vi "driveCheesy.vi"() -> ()   [LabVIEW 2012]
uses:
  <vilib>/Utility/inputDevices.llb/joystickAcquire.vi
panel:
  in  "low gear drive constant slow":dbl
  in  "low gear drive constant fast":dbl
  in  "Gear":bool
  in  "high gear drive constant slow":dbl
  in  "high gear drive constant fast":dbl
  in  "y axis":dbl
  in  "z axis":dbl
  out "Right Side Motors":dbl
  out "Left Side Motors":dbl
  # "High"
  # "Low"
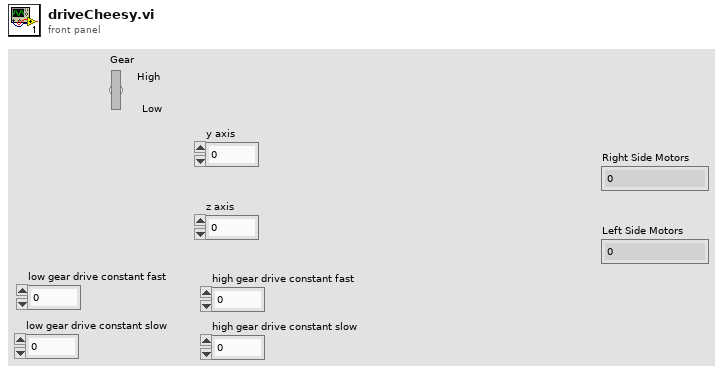
[diagram p1: front panel]
types:
  T1 = cluster{"X axis":i32, "Y axis":i32, "Z axis":i32, "X axis rotation":i32, "Y axis rotation":i32, "Z axis rotation":i32, "U axis":i32, "V axis":i32}
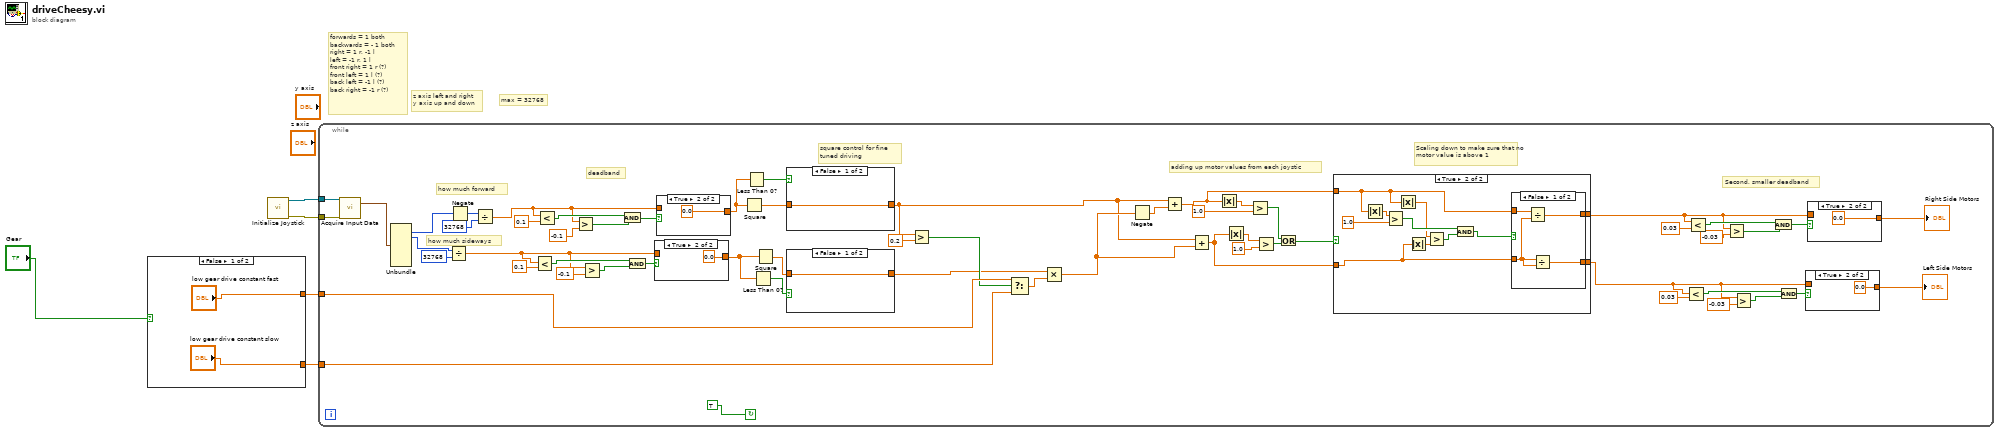
[diagram p0: block diagram]
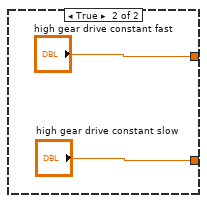
[diagram p2: hidden frame]
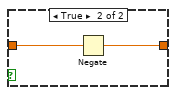
[diagram p3: hidden frame]
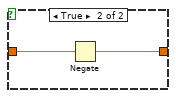
[diagram p4: hidden frame]
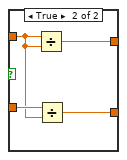
[diagram p10: hidden frame]
diagram:
  # "max = 32768"
  # "z axis left and right\ny axis up and down"
  # "forwards = 1 both\nbackwards = - 1 both\nright = 1 r, -1 l\nleft = -1 r, 1 l\nfront right = 1 r (?)\nfront left = 1 l (?)\nback left = -1 l (?)\nback right = -1 r (?)"
  n1 = case shown="False" "Gear" {
    tunnel: ["low gear drive constant fast" "high gear drive constant fast"] -> w3
    tunnel: ["low gear drive constant slow" "high gear drive constant slow"] -> w2
    frame False {
    }
    frame True {
    }
  }
  n2 = call <vilib>:"Initialize Joystick.vi"() -> ("error out"=w4:errorcluster, "device ID"=w5:refnum<k1>)  [unwired: 10 in]
  n3 = while {
    tunnel: w5 -> [w41]
    tunnel: w4 -> [w40]
    tunnel: w3 -> [w15]
    tunnel: w2 -> [w16]
    stop <- TRUE continue-if-true
    # "square control for fine tuned driving"
    # "Second, smaller deadband"
    # "Scaling down to make sure that no motor value is above 1"
    # "adding up motor values from each joystic"
    # "deadband"
    # "how much sideways"
    # "how much forward"
    n4 = call-poly <vilib>:"Acquire Input Data.vi"("device ID"=w41, "error in (no error)"=w40) -> ("axis info"=w39:T1)  [unwired: 13 in, 4 out]
    n5 = Unbundle(w39) -> ("Y axis"=w67:i32, "Z axis"=w38:i32)  [unwired: 6 out]
    n6 = Divide(x=w38, y=32768) -> (x/y=w52:dbl)
    n7 = Negate(x=w67) -> (-x=w66:i32)
    n8 = Divide(x=w66, y=32768) -> (x/y=w48:dbl)
    n9 = Less?(x=w52, y=0.1) -> (x < y?=w53:bool)
    n10 = Less?(x=w48, y=0.1) -> (x < y?=w49:bool)
    n11 = Greater?(x=w48, y=-0.1) -> (0:w46:bool)
    n12 = Greater?(x=w52, y=-0.1) -> (0:w50:bool)
    n13 = And(x=w49, y=w46) -> (x .and. y?=w55:bool)
    n14 = And(x=w53, y=w50) -> (x .and. y?=w54:bool)
    n15 = case shown="True" w54 {
      tunnel: [w79 0.0] -> w21
      tunnel: w52 -> [w79 _]
      frame False {
      }
      frame True {
      }
    }
    n16 = case shown="True" w55 {
      tunnel: [w81 0.0] -> w20
      tunnel: w48 -> [w81 _]
      frame False {
      }
      frame True {
      }
    }
    n17 = Square(x=w20) -> (x^2=w22:dbl)
    n18 = Less Than 0?(x=w20) -> (x < 0?=w25:bool)
    n19 = Less Than 0?(x=w21) -> (x < 0?=w24:bool)
    n20 = Square(x=w21) -> (x^2=w23:dbl)
    n21 = case shown="False" w25 {
      tunnel: w22 -> [w72 w74]
      tunnel: [w72 w73] -> w10
      frame False {
      }
      frame True {
        n22 = Negate(x=w74) -> (-x=w73:dbl)
      }
    }
    n23 = case shown="False" w24 {
      tunnel: w23 -> [w69 w70]
      tunnel: [w69 w71] -> w11
      frame False {
      }
      frame True {
        n24 = Negate(x=w70) -> (-x=w71:dbl)
      }
    }
    n25 = Greater?(x=w10, y=0.2) -> (0:w14:bool)
    n26 = Select(t=w15, s=w14, f=w16) -> (s? t:f=w12:dbl)
    n27 = Multiply(x=w11, y=w12) -> (x*y=w13:dbl)
    n28 = Negate(x=w13) -> (-x=w56:dbl)
    n29 = Add(x=w10, y=w56) -> (x+y=w43:dbl)
    n30 = Add(x=w10, y=w13) -> (x+y=w45:dbl)
    n31 = Absolute Value(x=w43) -> (abs(x)=w42:dbl)
    n32 = Absolute Value(x=w45) -> (abs(x)=w44:dbl)
    n33 = Greater?(x=w42, y=1.0) -> (0:w61:bool)
    n34 = Greater?(x=w44, y=1.0) -> (0:w60:bool)
    n35 = Or(x=w61, y=w60) -> (x .or. y?=w59:bool)
    n36 = case shown="True" w59 {
      tunnel: w43 -> [w84 w86]
      tunnel: w45 -> [w83 w88]
      tunnel: [w84 w94] -> w19
      tunnel: [w83 w93] -> w18
      frame False {
      }
      frame True {
        n37 = Absolute Value(x=w86) -> (abs(x)=w85:dbl)
        n38 = Greater?(x=w85, y=1.0) -> (0:w92:bool)
        n39 = Absolute Value(x=w86) -> (abs(x)=w87:dbl)
        n40 = Absolute Value(x=w88) -> (abs(x)=w89:dbl)
        n41 = Greater?(x=w87, y=w89) -> (0:w90:bool)
        n42 = And(x=w92, y=w90) -> (x .and. y?=w91:bool)
        n43 = case shown="False" w91 {
          tunnel: w86 -> [w99 w100]
          tunnel: w88 -> [w97 w103]
          tunnel: [w98 w102] -> w94
          tunnel: [w96 w101] -> w93
          frame False {
            n44 = Divide(x=w99, y=w97) -> (x/y=w98:dbl)
            n45 = Divide(x=w97, y=w97) -> (x/y=w96:dbl)
          }
          frame True {
            n46 = Divide(x=w100, y=w100) -> (x/y=w102:dbl)
            n47 = Divide(x=w103, y=w100) -> (x/y=w101:dbl)
          }
        }
      }
    }
    n48 = Less?(x=w18, y=0.03) -> (x < y?=w32:bool)
    n49 = Less?(x=w19, y=0.03) -> (x < y?=w35:bool)
    n50 = Greater?(x=w19, y=-0.03) -> (0:w37:bool)
    n51 = Greater?(x=w18, y=-0.03) -> (0:w34:bool)
    n52 = And(x=w35, y=w37) -> (x .and. y?=w30:bool)
    n53 = And(x=w32, y=w34) -> (x .and. y?=w31:bool)
    n54 = case shown="True" w31 {
      tunnel: [w75 0.0] -> w27
      tunnel: w18 -> [w75 _]
      frame False {
      }
      frame True {
      }
    }
    "Left Side Motors" <- w27
    n55 = case shown="True" w30 {
      tunnel: [w77 0.0] -> w26
      tunnel: w19 -> [w77 _]
      frame False {
      }
      frame True {
      }
    }
    "Right Side Motors" <- w26
  }
